vi "EnQueue_Message_Multiple.vi"(6 "Priority Message? Array":bool[](array[boolean]), 8 "error in (no error)":errorcluster, 9 "Message Data Array":variant[](array[variant]), 10 "Message Array":string[](array[string]), 11 "Message_Queue":refnum<queue>) -> (0 "error out":errorcluster, 3 "Dup_Message_Queue":refnum<queue>)   [LabVIEW 2014]
uses:
  02_Controls/Message_Data_Ctl.ctl
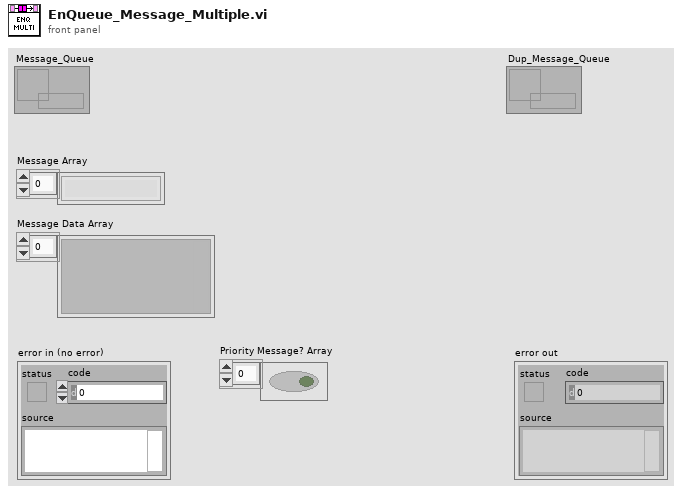
[diagram p1: front panel]
types:
  T1 = typedef "Message_Data_Ctl.ctl" = cluster{"Message":string, "Data":variant}
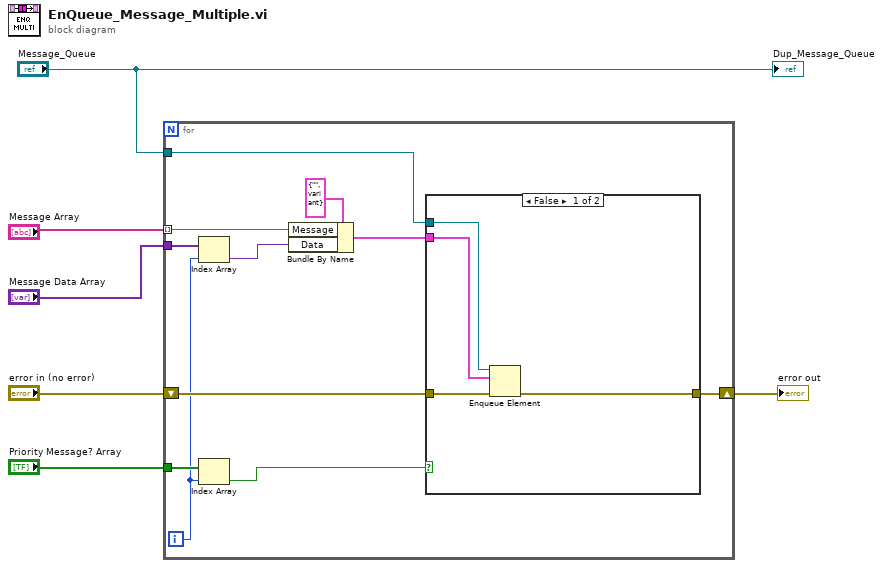
[diagram p0: block diagram]
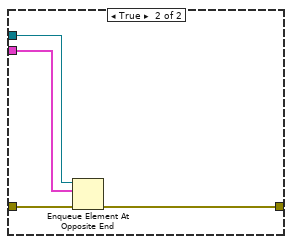
[diagram p2: hidden frame]
diagram:
  n1 = for {
    tunnel: "Message Array" -> [w17] mode=indexing
    tunnel: "Message Data Array" -> [w12]
    tunnel: "Priority Message? Array" -> [w10]
    tunnel: "Message_Queue" -> [w14]
    shift-right: [w15] -> w2
    shift-left: "error in (no error)" -> [w16]
    i -> [w8]
    n2 = Index Array(array=w12, index=w8) -> (element=w11:variant)
    n3 = Index Array(array=w10, index=w8) -> (element=w9:bool)
    n4 = Bundle By Name(cluster=T1 {"Message"="", "Data"=variant} ("Message_Data"), "Message"=w17, "Data"=w11) -> (w13:T1)
    n5 = case shown="False" w9 {
      tunnel: w16 -> [w21 w25]
      tunnel: [w20 w24] -> w15
      tunnel: w14 -> [w19 w23]
      tunnel: w13 -> [w18 w22]
      frame False {
        n6 = Enqueue Element(queue=w19, element=w18, error in (no error)=w21) -> (error out=w20:errorcluster)  [unwired: 1 in, 2 out]
      }
      frame True {
        n7 = Enqueue Element At Opposite End(queue=w23, element=w22, error in (no error)=w25) -> (error out=w24:errorcluster)  [unwired: 1 in, 2 out]
      }
    }
  }
  "error out" <- w2
  "Dup_Message_Queue" <- "Message_Queue"
